vi "Motor Errors.vi"() -> ()   [LabVIEW 2012]
panel:
  in  "Front Right Steer":dbl
  in  "Front Left Steer":dbl
  in  "Rear Right Steer":dbl
  in  "Rear Left Steer":dbl
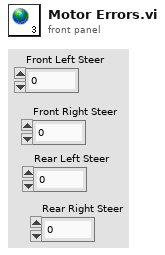
[diagram p1: front panel]
diagram:
